vi "sub_remove_DMD_mov.vi"(2 "SequenceId":u32, 3 "DeviceId":u32) -> (0 "SeqFreeErr":i32, 1 "DevFreeErr":i32)   [LabVIEW 2013]
uses:
  C:/Program Files/ALP-4.1/ALP-4.1 high-speed API/Samples/alpD41.dll
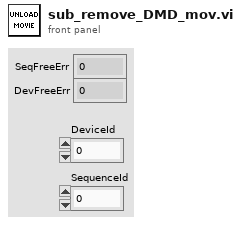
[diagram p1: front panel]
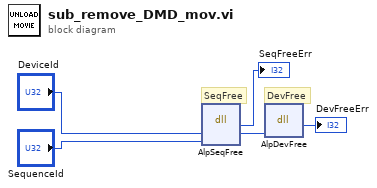
[diagram p0: block diagram]
diagram:
  # "DevFree"
  # "SeqFree"
  n1 = dll-call lib="C:/Program Files/ALP-4.1/ALP-4.1 high-speed API/Samples/alpD41.dll" fn="AlpSeqFree"("DeviceId"="DeviceId", "SequenceId"="SequenceId") -> ("return type"=→"SeqFreeErr":i32, "DeviceId"=w5:u32)  [unwired: 4 in, 2 out]
  n2 = dll-call lib="C:/Program Files/ALP-4.1/ALP-4.1 high-speed API/Samples/alpD41.dll" fn="AlpDevFree"("DeviceId"=w5) -> ("return type"=→"DevFreeErr":i32)  [unwired: 4 in, 2 out]
